vi "LS372Monitor.vi"() -> ()   [LabVIEW 2016]
uses:
  Instrument_Setup.vi
  Global/Global Variables/Data_Display_global.vi
  Equipment/Lake Shore 372/Lake Shore 372.lvlib
panel:
  in  "Stopp":bool
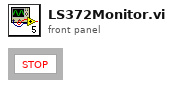
[diagram p1: front panel]
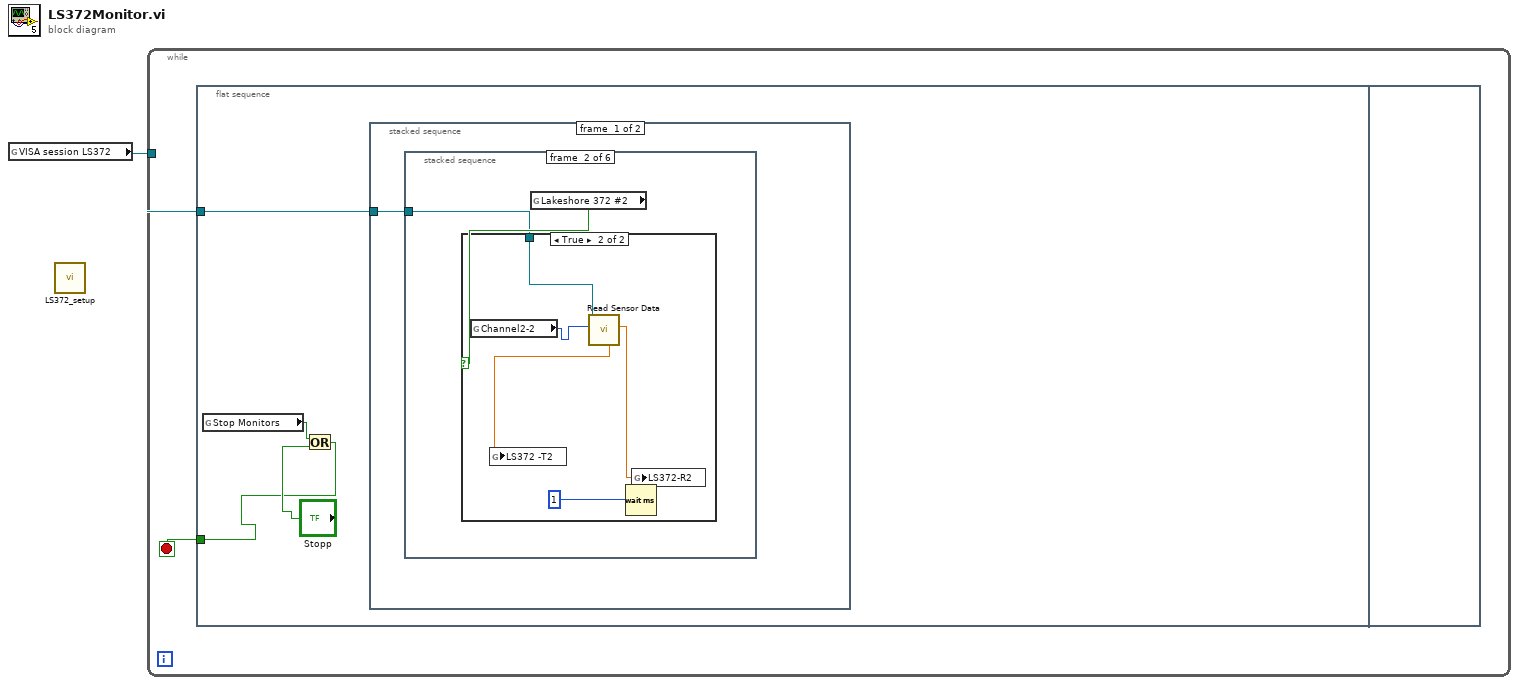
[diagram p0: block diagram]
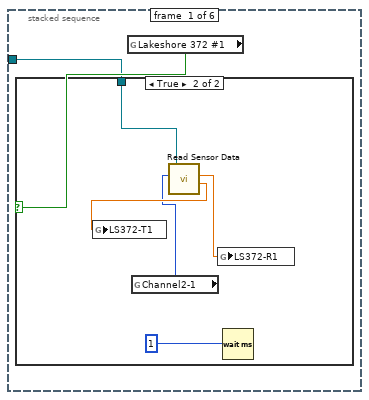
[diagram p2: hidden frame]
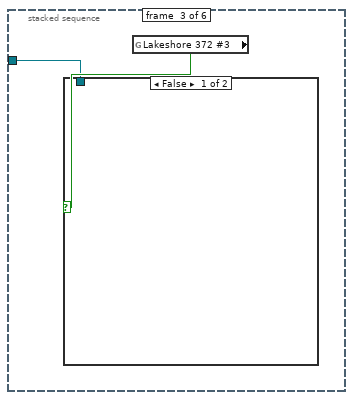
[diagram p5: hidden frame]
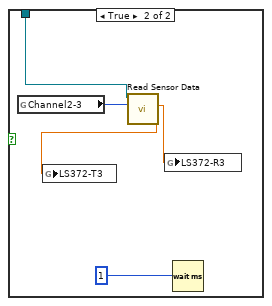
[diagram p6: hidden frame]
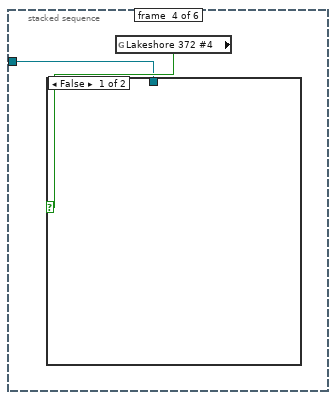
[diagram p7: hidden frame]
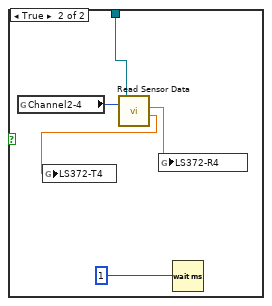
[diagram p8: hidden frame]
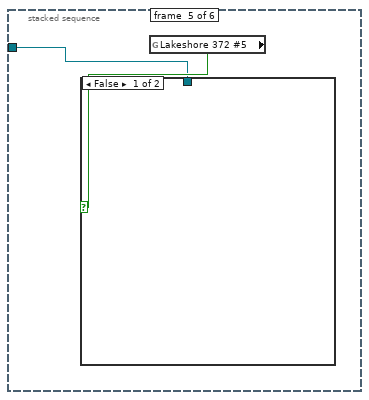
[diagram p9: hidden frame]
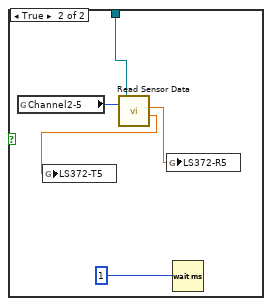
[diagram p10: hidden frame]
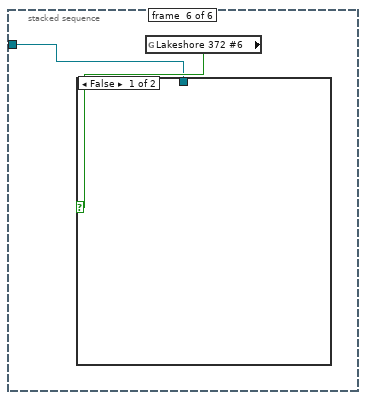
[diagram p11: hidden frame]
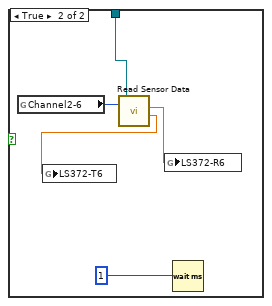
[diagram p12: hidden frame]
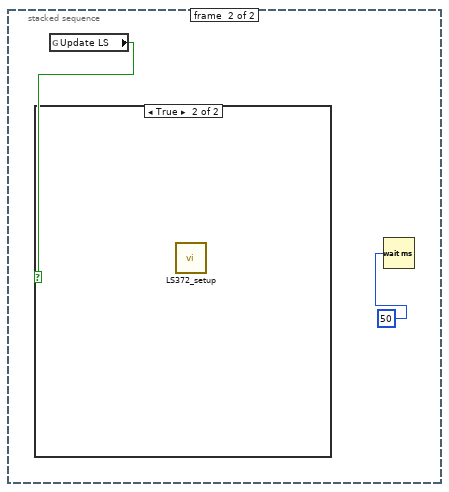
[diagram p13: hidden frame]
diagram:
  n1 = global read "Instrument_Setup.vi" "VISA session LS372"() -> (w1:refnum<visa-resource-name>)
  n2 = call "LS372_setup.vi"() -> ()  [unwired: 1 in]
  n3 = while {
    tunnel: w1 -> [w2]
    stop <- w3 stop-if-true
    n4 = flat-sequence {
      tunnel: [w4] -> w3
      tunnel: w2 -> [w7]
      frame #0 {
        n5 = global read "Data_Display_global.vi" "Stop Monitors"() -> (w6:bool)
        n6 = Or(x=w6, y="Stopp") -> (x .or. y?=w4:bool)
        n7 = stacked-sequence {
          tunnel: w7 -> [w8 _]
          frame #0 {
            n8 = stacked-sequence {
              tunnel: w8 -> [w9 w16 w23 w30 w37 w44]
              frame #0 {
                n9 = global read "Instrument_Setup.vi" "Lakeshore 372 #1"() -> (w10:bool)
                n10 = case shown="True" w10 {
                  tunnel: w9 -> [_ w13]
                  frame False {
                  }
                  frame True {
                    n11 = global read "Instrument_Setup.vi" "Channel2-1"() -> (w11:u16)
                    n12 = call "Read Sensor Data.vi"("Channel (1:1)"=w11, "VISA resource name"=w13) -> ("Kelvin Reading"=w12:dbl, "Resistance Reading"=w14:dbl)  [unwired: 4 in, 4 out]
                    n13 = global write "Data_Display_global.vi" "LS372-T1"(w12) -> ()
                    n14 = global write "Data_Display_global.vi" "LS372-R1"(w14) -> ()
                    n15 = Wait (ms)(milliseconds to wait=1) -> ()  [unwired: 1 out]
                  }
                }
              }
              frame #1 {
                n16 = global read "Instrument_Setup.vi" "Lakeshore 372 #2"() -> (w17:bool)
                n17 = case shown="True" w17 {
                  tunnel: w16 -> [_ w21]
                  frame False {
                  }
                  frame True {
                    n18 = global read "Instrument_Setup.vi" "Channel2-2"() -> (w18:u16)
                    n19 = call "Read Sensor Data.vi"("Channel (1:1)"=w18, "VISA resource name"=w21) -> ("Kelvin Reading"=w19:dbl, "Resistance Reading"=w20:dbl)  [unwired: 4 in, 4 out]
                    n20 = global write "Data_Display_global.vi" "LS372 -T2"(w19) -> ()
                    n21 = Wait (ms)(milliseconds to wait=1) -> ()  [unwired: 1 out]
                    n22 = global write "Data_Display_global.vi" "LS372-R2"(w20) -> ()
                  }
                }
              }
              frame #2 {
                n23 = global read "Instrument_Setup.vi" "Lakeshore 372 #3"() -> (w24:bool)
                n24 = case shown="False" w24 {
                  tunnel: w23 -> [_ w27]
                  frame False {
                  }
                  frame True {
                    n25 = global read "Instrument_Setup.vi" "Channel2-3"() -> (w25:u16)
                    n26 = call "Read Sensor Data.vi"("Channel (1:1)"=w25, "VISA resource name"=w27) -> ("Kelvin Reading"=w26:dbl, "Resistance Reading"=w28:dbl)  [unwired: 4 in, 4 out]
                    n27 = global write "Data_Display_global.vi" "LS372-T3"(w26) -> ()
                    n28 = global write "Data_Display_global.vi" "LS372-R3"(w28) -> ()
                    n29 = Wait (ms)(milliseconds to wait=1) -> ()  [unwired: 1 out]
                  }
                }
              }
              frame #3 {
                n30 = global read "Instrument_Setup.vi" "Lakeshore 372 #4"() -> (w31:bool)
                n31 = case shown="False" w31 {
                  tunnel: w30 -> [_ w33]
                  frame False {
                  }
                  frame True {
                    n32 = global read "Instrument_Setup.vi" "Channel2-4"() -> (w32:u16)
                    n33 = call "Read Sensor Data.vi"("Channel (1:1)"=w32, "VISA resource name"=w33) -> ("Kelvin Reading"=w35:dbl, "Resistance Reading"=w34:dbl)  [unwired: 4 in, 4 out]
                    n34 = global write "Data_Display_global.vi" "LS372-T4"(w35) -> ()
                    n35 = global write "Data_Display_global.vi" "LS372-R4"(w34) -> ()
                    n36 = Wait (ms)(milliseconds to wait=1) -> ()  [unwired: 1 out]
                  }
                }
              }
              frame #4 {
                n37 = global read "Instrument_Setup.vi" "Lakeshore 372 #5"() -> (w38:bool)
                n38 = case shown="False" w38 {
                  tunnel: w37 -> [_ w40]
                  frame False {
                  }
                  frame True {
                    n39 = global read "Instrument_Setup.vi" "Channel2-5"() -> (w39:u16)
                    n40 = call "Read Sensor Data.vi"("Channel (1:1)"=w39, "VISA resource name"=w40) -> ("Kelvin Reading"=w42:dbl, "Resistance Reading"=w41:dbl)  [unwired: 4 in, 4 out]
                    n41 = global write "Data_Display_global.vi" "LS372-T5"(w42) -> ()
                    n42 = global write "Data_Display_global.vi" "LS372-R5"(w41) -> ()
                    n43 = Wait (ms)(milliseconds to wait=1) -> ()  [unwired: 1 out]
                  }
                }
              }
              frame #5 {
                n44 = global read "Instrument_Setup.vi" "Lakeshore 372 #6"() -> (w45:bool)
                n45 = case shown="False" w45 {
                  tunnel: w44 -> [_ w47]
                  frame False {
                  }
                  frame True {
                    n46 = global read "Instrument_Setup.vi" "Channel2-6"() -> (w46:u16)
                    n47 = call "Read Sensor Data.vi"("Channel (1:1)"=w46, "VISA resource name"=w47) -> ("Kelvin Reading"=w49:dbl, "Resistance Reading"=w48:dbl)  [unwired: 4 in, 4 out]
                    n48 = global write "Data_Display_global.vi" "LS372-T6"(w49) -> ()
                    n49 = global write "Data_Display_global.vi" "LS372-R6"(w48) -> ()
                    n50 = Wait (ms)(milliseconds to wait=1) -> ()  [unwired: 1 out]
                  }
                }
              }
            }
          }
          frame #1 {
            n51 = global read "Data_Display_global.vi" "Update LS"() -> (w51:bool)
            n52 = case shown="True" w51 {
              frame False {
              }
              frame True {
                n53 = call "LS372_setup.vi"() -> ()  [unwired: 1 in]
              }
            }
            n54 = Wait (ms)(milliseconds to wait=50) -> ()  [unwired: 1 out]
          }
        }
      }
      frame #1 {
      }
    }
  }
